vi "Disconnect.vi"(8 "error in":errorcluster, 11 "6032A in":refnum<class "6032A.lvclass">) -> (0 "error out":errorcluster, 3 "6032A out":refnum<class "6032A.lvclass">)   [LabVIEW 2019, in "6032A.lvlib" / "6032A.lvclass"]
doc: "This disconnect routine is a must override from the Instrument Class\nChildren Classes are responsible for handling the override, but the parent class is an intermediary and must contain the override functions to maintain the rules for the method."
uses:
  Library/6032A.lvclass
  Library/6032A.lvclass/6032A.ctl
  builds/Instruments/PowerSupply.lvlibp/Library/PowerSupply.lvclass
  <instrlib>/Agilent 6XXX Series/Agilent 6XXX Series.lvlib
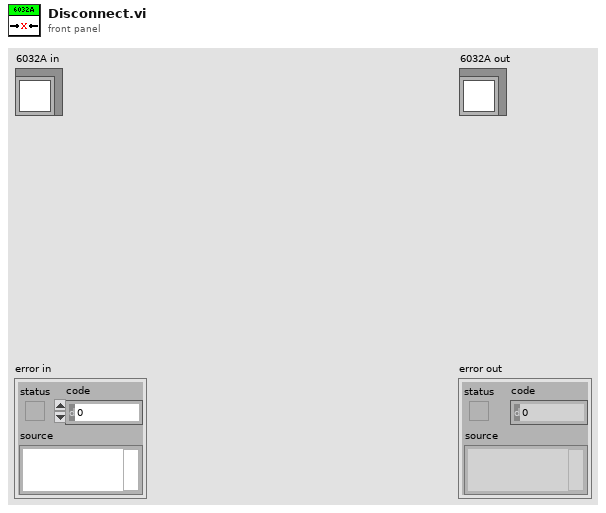
[diagram p1: front panel]
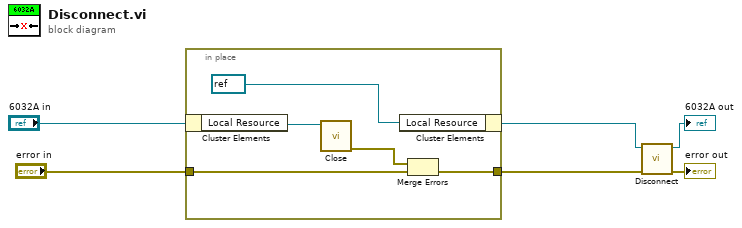
[diagram p0: block diagram]
diagram:
  n1 = in-place {
    in-place-border: "error in" -> [w7]
    in-place-border: [w8] -> w1
    n2 = in-place-cluster #1("6032A in") -> ("Local Resource"=w11:refnum<visa-resource-name>)
    n3 = call <instrlib>:"Close.vi"("VISA resource name"=w11) -> ("error out"=w9:errorcluster)  [unwired: 10 in]
    n4 = in-place-cluster #1("Local Resource"=refnum<visa-resource-name> refnum) -> (w3:refnum<class "6032A.lvclass">)
    n5 = Merge Errors(w9, w7) -> (w8:errorcluster)
  }
  n6 = call-parent "Disconnect.vi"("error in"=w1, "PowerSupply in"=w3) -> ("error out"=→"error out":errorcluster, "PowerSupply out"=→"6032A out":refnum<class "6032A.lvclass">)  [unwired: 8 in]
